vi "Data extraction from Graph.vi"(11 "Test Graph1 2":cluster{"Horz Time array":dbl[], "Y":dbl[]}[](graph) caption="C2-RX4 Differential Impedance") -> (3 "Data out":dbl[][](array[numeric]))   [LabVIEW 2011]
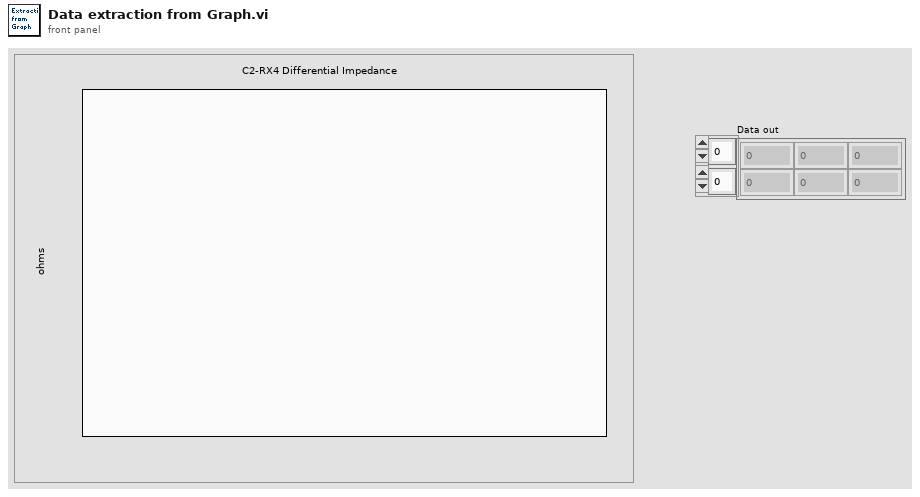
[diagram p1: front panel]
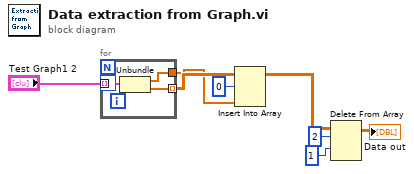
[diagram p0: block diagram]
diagram:
  n1 = for "For循环" {
    tunnel: "Test Graph1 2" -> [w11] mode=indexing
    tunnel: [w10] -> w7 mode=indexing
    tunnel: [w9] -> w6
    workers-P: _ -> [_]
    n2 = Unbundle(w11) -> ("Horz Time array"=w9:dbl[], "Y"=w10:dbl[])
  }
  n3 = Insert Into Array(array=w7, index (row)=0 ("索引 (行)"), new element=w6) -> (w4:dbl[][])  [unwired: 1 in]
  n4 = Delete From Array(array=w4, length=2 ("长度"), index (row)=1 ("索引 (行)")) -> (array with subset deleted=→"Data out":dbl[][])  [unwired: 1 in, 1 out]
